vi "PFI-28000-Base_Set Overloads.vi"(8 "error in (no error)":errorcluster, 10 "Overloads":refnum<data-value>, 11 "PFI-28000-Base in":refnum<class "PFI-28000-Base.lvclass">) -> (0 "error out":errorcluster, 3 "PFI-28000-Base out":refnum<class "PFI-28000-Base.lvclass">)   [LabVIEW 2017, in "PFI-28000-Base.lvclass"]
uses:
  PFI-28000-Base.lvclass
  PFI-28000-Base.lvclass/PFI-28000-Base.ctl
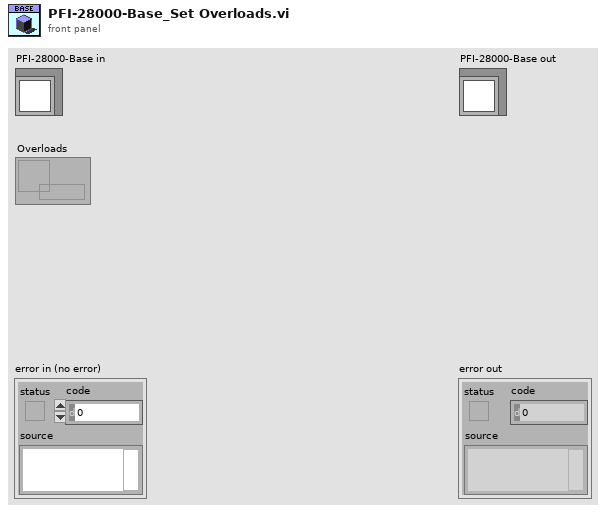
[diagram p1: front panel]
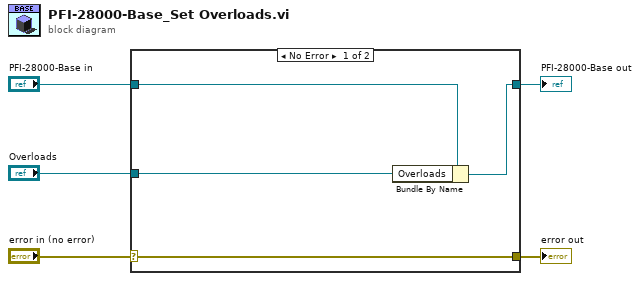
[diagram p0: block diagram]
diagram:
  n1 = case shown="No Error" "error in (no error)" {
    selector: "error in (no error)" -> [w9 w10]
    tunnel: [w9 w10] -> w4
    tunnel: [w7 w11] -> w2
    tunnel: "PFI-28000-Base in" -> [w8 w11]
    tunnel: "Overloads" -> [w6 _]
    frame No Error {
      n2 = Bundle By Name(cluster=w8, "Overloads"=w6) -> (w7:refnum<class "PFI-28000-Base.lvclass">)
    }
    frame Error {
    }
  }
  "error out" <- w4
  "PFI-28000-Base out" <- w2
